vi "Get Node Reference.vi"(8 "error in":errorcluster, 11 "Node Ptr":T1 format="%.0x") -> (0 "error out":errorcluster, 2 "BaseNodeType":refnum<k24>, 3 "Node Ptr":T1 format="%.0x", 4 "Base Node":refnum<k24>)   [LabVIEW 2026]
uses:
  <vilib>/NI VeriStand/Custom Device API/Custom Device Item Ref.ctl
  NationalInstruments.VeriStand.SystemStorage
  NationalInstruments.VeriStand.SystemDefinitionAPI
  <vilib>/NI VeriStand/Custom Device API/Custom Device API.lvlib
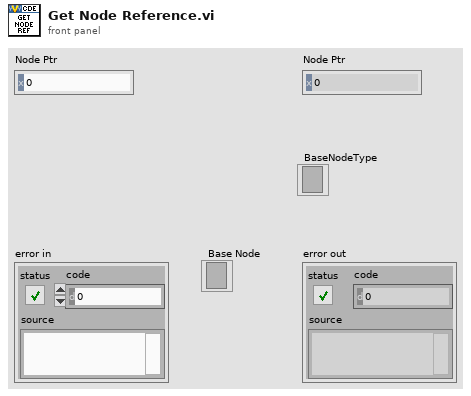
[diagram p1: front panel]
types:
  T1 = typedef "Custom Device API.lvlib/Custom Device Item Ref.ctl" = u64
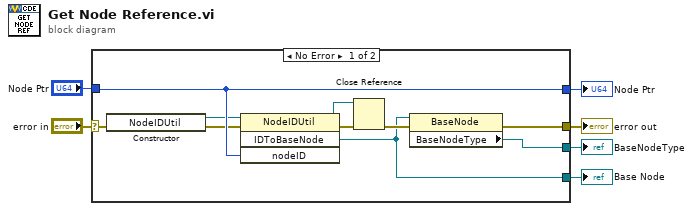
[diagram p0: block diagram]
diagram:
  n1 = case shown="No Error" "error in" {
    selector: "error in" -> [w16 w18]
    tunnel: [w8 w18] -> w5
    tunnel: [w15 _] -> w4
    tunnel: "Node Ptr" -> [w14 w17]
    tunnel: [w14 w17] -> w2
    tunnel: [w7 _] -> w1
    frame No Error {
      n2 = constructor class="NodeIDUtil"(error in=w16) -> (reference out=w9:refnum<k24>, error out=w11:errorcluster)  [unwired: 2 in, 1 out]
      n3 = invoke class="NodeIDUtil" method="IDToBaseNode"(reference=w9, error in=w11, "nodeID"=w14) -> (reference out=w10:refnum<k24>, error out=w12:errorcluster, "IDToBaseNode"=w7:refnum<k24>)  [unwired: 1 in, 1 out]
      n4 = Close Reference(reference=w10, error in (no error)=w12) -> (error out=w13:errorcluster)
      n5 = property class="BaseNode"(reference=w7, error in=w13) -> (error out=w8:errorcluster, "BaseNodeType"=w15:refnum<k24>)  [unwired: 1 out]
    }
    frame Error {
    }
  }
  "error out" <- w5
  "BaseNodeType" <- w4
  "Node Ptr" <- w2
  "Base Node" <- w1
